vi "Multitone Waveform.vi"() -> ()   [LabVIEW 2014]
doc: "Shows how to configure then create an arbitrary waveform."
uses:
  Instance           1 56Saved   Agilent 33XXX Series Generate Arbitrary Waveform .vi
  Instance           2 56Saved   Agilent 33XXX Series Generate Arbitrary Waveform .vi
  Agilent 33XXX Series/Agilent 33XXX Series.lvlib
  <vilib>/measure/NI_MAPro.lvlib
  <vilib>/measure/NI_MABase.lvlib
panel:
  in  "signal type":T1(ring)
  out "Waveform Graph":dbl[](graph)
  in  "OK Button":bool
  in  "MT params":T2={"tone frequencies"=[1.0, 0.0, 0.0, 0.0], "tone amplitudes"=[1.0, 0.0, 0.0, 0.0], "tone phases"=[0.0, 0.0, 0.0, 0.0]} {"tone phases" format="%.2p"; "tone amplitudes" format="%.2p"; "tone frequencies" format="%.2p"}
  in  "Ring":u16(ring) items=["Multitone", "Arbitrary"]
  in  "sampling info":cluster{"Fs":dbl, "#s":dbl}={"Fs"=14400.0, "#s"=14400.0} {"Fs" format="%.2p"}
  in  "Serial Configuration":T3={"Baud Rate"=9600, "Parity"=0, "Data Bits"=8, "Flow Control"=4} {"Flow Control" items=["None", "XON/XOFF", "RTS/CTS", "XON/XOFF & RTS/CTS", "DTR/DSR", "XON/XOFF & DTR/DSR"]; "Data Bits" items=["7"=7, "8"=8]; "Parity" items=["None", "Odd", "Even", "Mark", "Space"]; "Baud Rate" items=["300"=300, "600"=600, "1200"=1200, "2400"=2400, "4800"=4800, "9600"=9600, "19200"=19200]}
  in  "VISA resource name":refnum<visa-resource-name>="GPIB0::15::INSTR"
  in  "Frequency (Hz)":dbl=50.0
  in  "Amplitude (V)":dbl=5.0
  in  "Offset (0 V)":dbl
  in  "Arbitrary Waveform Name":string="ARB1"
  # "(c) 2005 - 2013 National Instruments.  ALL RIGHTS RESERVED."
  # "To edit the Arbitrary Waveform, use the Simulate Arbitrary Signal on the block diagram."
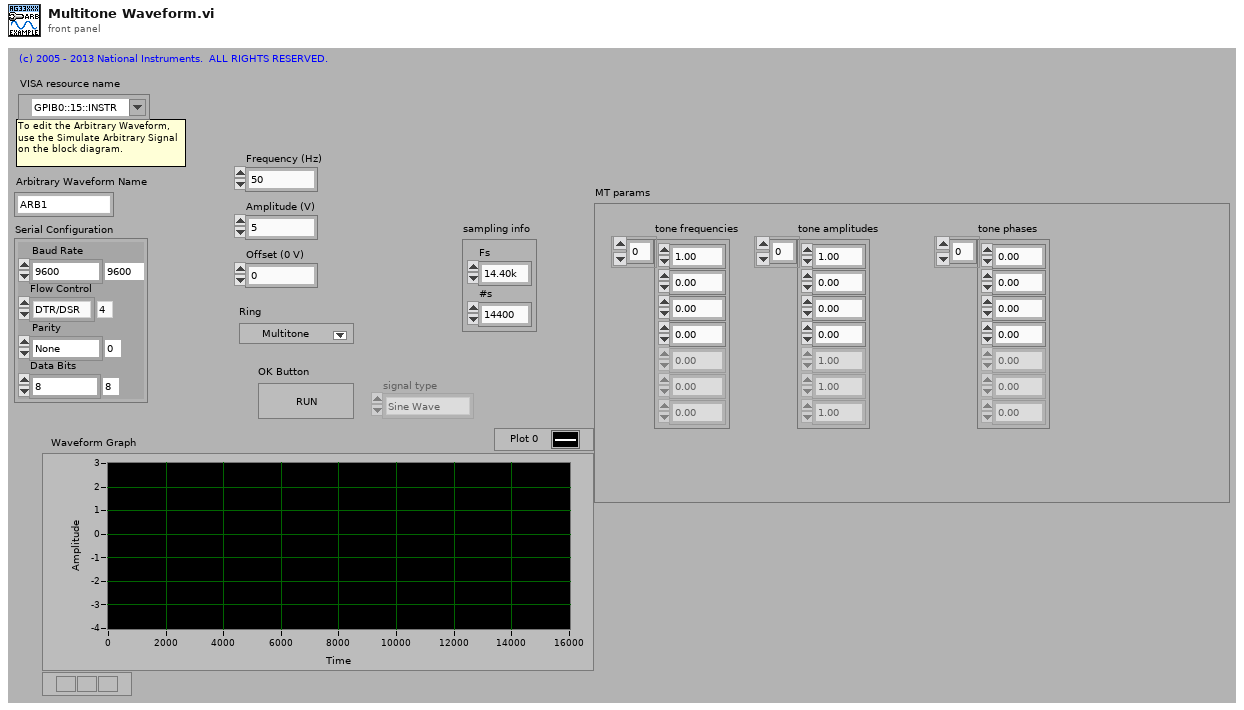
[diagram p1: front panel]
types:
  T1 = enum16{"Sine Wave", "Triangle Wave", "Square Wave", "Sawtooth Wave"}
  T2 = cluster{"tone frequencies":dbl[], "tone amplitudes":dbl[], "tone phases":dbl[]}
  T3 = cluster{"Baud Rate":u32, "Parity":u16, "Data Bits":u16, "Flow Control":u16}
  T4 = enum8{"Enabled", "Disabled", "Disabled and Grayed Out"}
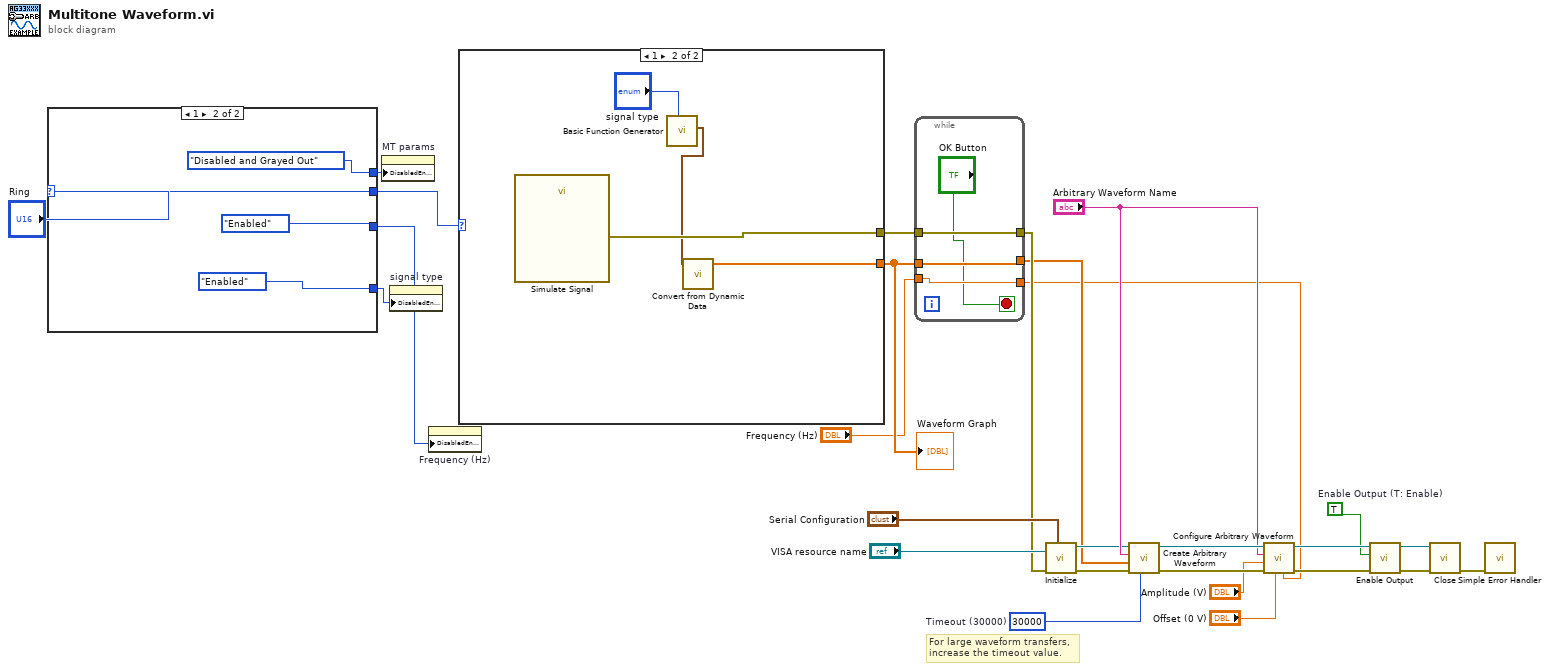
[diagram p0: block diagram]
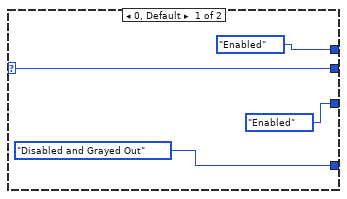
[diagram p2: hidden frame]
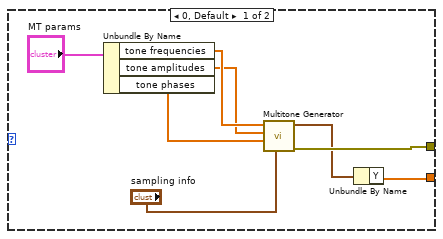
[diagram p3: hidden frame]
diagram:
  w16 = u32 30000  # Timeout (30000)
  w20 = TRUE  # Enable Output (T: Enable)
  # "For large waveform transfers, increase the timeout value."
  n1 = case shown="1" "Ring" {
    selector: "Ring" -> [w29 w33]
    tunnel: [T4."Enabled" ("Disabled") T4."Disabled and Grayed Out" ("Disabled")] -> w10
    tunnel: [T4."Enabled" ("Disabled") T4."Enabled" ("Disabled")] -> w9
    tunnel: [w29 w33] -> w8
    tunnel: [T4."Disabled and Grayed Out" ("Disabled") T4."Enabled" ("Disabled")] -> w1
    frame 0, Default {
    }
    frame 1 {
    }
  }
  n2 = property on="MT params" class="Clust (strict)"("DisabledEnum"=w10) -> ()  [unwired: 2 in, 2 out]
  n3 = property on="signal type" class="Enum (strict)"("DisabledEnum"=w1) -> ()  [unwired: 2 in, 2 out]
  n4 = property on="Frequency (Hz)" class="DigNum (strict)"("DisabledEnum"=w9) -> ()  [unwired: 2 in, 2 out]
  n5 = case shown="1" w8 {
    tunnel: [w36 w47] -> w3
    tunnel: [w43 w46] -> w7
    frame 0, Default {
      n6 = Unbundle By Name("MT params") -> ("tone frequencies"=w40:dbl[], "tone amplitudes"=w39:dbl[], "tone phases"=w38:dbl[])
      n7 = call <vilib>:"Multitone Generator.vi"("sampling info"="sampling info", "tone phases"=w38, "tone amplitudes"=w39, "tone frequencies"=w40) -> ("error out"=w43:errorcluster, "signal out"=w37:waveform(dbl))  [unwired: 4 in, 2 out]
      n8 = Unbundle By Name(w37) -> ("Y"=w36:dbl[])
    }
    frame 1 {
      n9 = call "Simulate Signal"() -> ("error out"=w46:errorcluster)  [unwired: 14 in, 1 out]
      n10 = call <vilib>:"Basic Function Generator.vi"("signal type"="signal type") -> ("signal out"=w44:waveform(dbl))  [unwired: 8 in, 2 out]
      n11 = call "Convert from Dynamic Data"("Dynamic Data Type"=w44) -> ("Array"=w47:dbl[])  [unwired: 3 in]
    }
  }
  "Waveform Graph" <- w3
  n12 = while {
    tunnel: w7 -> [w51]
    tunnel: [w51] -> w6
    tunnel: [w50] -> w5
    tunnel: w3 -> [w50]
    tunnel: [w49] -> w4
    tunnel: "Frequency (Hz)" -> [w49]
    stop <- "OK Button" stop-if-true
  }
  n13 = call "Initialize.vi"("Serial Configuration"="Serial Configuration", "error in (no error)"=w6, "VISA resource name"="VISA resource name") -> ("error out"=w14:errorcluster, "VISA resource name out"=w15:refnum<visa-resource-name>)  [unwired: 7 in]
  n14 = call "Create Arbitrary Waveform.vi"("Timeout (10000)"=w16, "error in (no error)"=w14, "Arbitrary Waveform Data"=w5, "Arbitrary Waveform Name (\"ARB1\")"="Arbitrary Waveform Name", "VISA resource name"=w15) -> ("error out"=w25:errorcluster, "VISA resource name out"=w26:refnum<visa-resource-name>)  [unwired: 5 in]
  n15 = call "Configure Arbitrary Waveform.vi"("Frequency (1000 Hz)"=w4, "Offset (0.00 V)"="Offset (0 V)", "error in (no error)"=w25, "Gain (1.0)"="Amplitude (V)", "Arbitrary Waveform Name (\"ARB1\")"="Arbitrary Waveform Name", "VISA resource name"=w26) -> ("error out"=w23:errorcluster, "VISA resource name out"=w24:refnum<visa-resource-name>)  [unwired: 4 in]
  n16 = call "Enable Output.vi"("error in (no error)"=w23, "Enable Output  (T: Enable)"=w20, "VISA resource name"=w24) -> ("error out"=w22:errorcluster, "VISA resource name out"=w21:refnum<visa-resource-name>)  [unwired: 7 in]
  n17 = call "Close.vi"("error in (no error)"=w22, "VISA resource name"=w21) -> ("error out"=w27:errorcluster)  [unwired: 9 in]
  n18 = call <vilib>:"Simple Error Handler.vi"("error in (no error)"=w27) -> ()  [unwired: 4 in, 5 out]
